vi "Tusk.Test.vi"(10 "Tusk in":refnum<class "Tusk.lvclass">) -> ()   [LabVIEW 2018, in "Application.lvlib" / "Tusk.lvclass"]
uses:
  Tusk.lvclass
  Tusk.lvclass/Tusk.ctl
  Store Class/Store.lvclass/Store.ctl
  Dictionary Class/Dictionary.lvclass/Dictionary.ctl
  Message Class/Message.lvclass/Message.ctl
  Tusk.ValidateName.vi
  Tusk.SetName (Global).vi
  Store Class/VIs/Create.vi
  Tusk.GetName (Global).vi
  Store Class/VIs/Destroy.vi
  Tusk.Init.vi
  Tusk.Register.vi
  Tusk.ValidateTusk (Local).vi
  Tusk.SetName (Local).vi
  Message Class/VIs/Wrap Message.vi
  Tusk.GetName (Local).vi
  Keywords Class/VIs/{Timeout}.vi
  Keywords Class/VIs/{Destructor}.vi
  Tusk.IsGlogalMessage.vi
  Tusk.MessageSenderCore.vi
  Tusk.GetTuskFromDictionary.vi
  Message Class/VIs/Split Message.vi
  Message Class/VIs/Get Message.vi
  Tusk.IsTopLevel.vi
  Tusk.KillAll(Local).vi
  Message Class/VIs/Unwrap Message.vi
  Keywords Class/VIs/{Self}.vi
  Tusk.KillMessageCore.vi
  Exceptions Class/VIs/Invalid Name Format.vi
  Keywords Class/VIs/{Constructor}.vi
  Tusk.GetDictionary.vi
  Tusk.Register.vi/ecdc04cd-daca-4470-8ca9-75b19434ba98.vi
  Dictionary Class/VIs/Get.vi
  Exceptions Class/VIs/Name (Local) Taken.vi
  Exceptions Class/VIs/Invalid Type.vi
  Tusk.GetTuskFromDictionary.vi/3fa77438-33e4-48e7-a501-c74b9750b9f8.vi
  Tusk.GetTuskFromDictionary.vi/bb4b4b2f-5120-4767-9776-c61ed956de36.vi
  Tusk.MessageAllSenderCore.vi
  Keywords Class/VIs/{All}.vi
  Dictionary Class/VIs/Get Data DVR.vi
  Tusk.MessageAllSenderCore.vi/1679c56e-e765-44f0-aff8-f47c4dbf3d60.vi
  <vilib>/Utility/error.llb/Trim Whitespace.vi
  Dictionary Class/VIs/Create.vi
  Dictionary Class/VIs/Destroy.vi
  Tusk.TuskBox.vi
  <vilib>/Utility/error.llb/Error Cluster From Error Code.vi
  <vilib>/Utility/SystemLogging/Write to System Log.vi
  Store Class/Store.lvclass
  Dictionary Class/Dictionary.lvclass
  Message Class/Message.lvclass
panel:
  out "x-y":dbl format="%^#_6e"
  out "Recieved Message":string
  in  "Send":bool
  in  "Message":string="Hello World!"
  in  "stop":bool
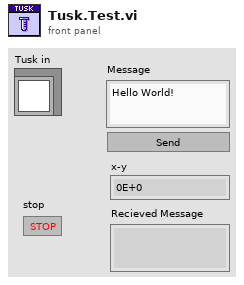
[diagram p1: front panel]
types:
  T1 = typedef "Application.lvlib/Message.lvclass/Event Registration Refnum.ctl" = refnum<event-registration>
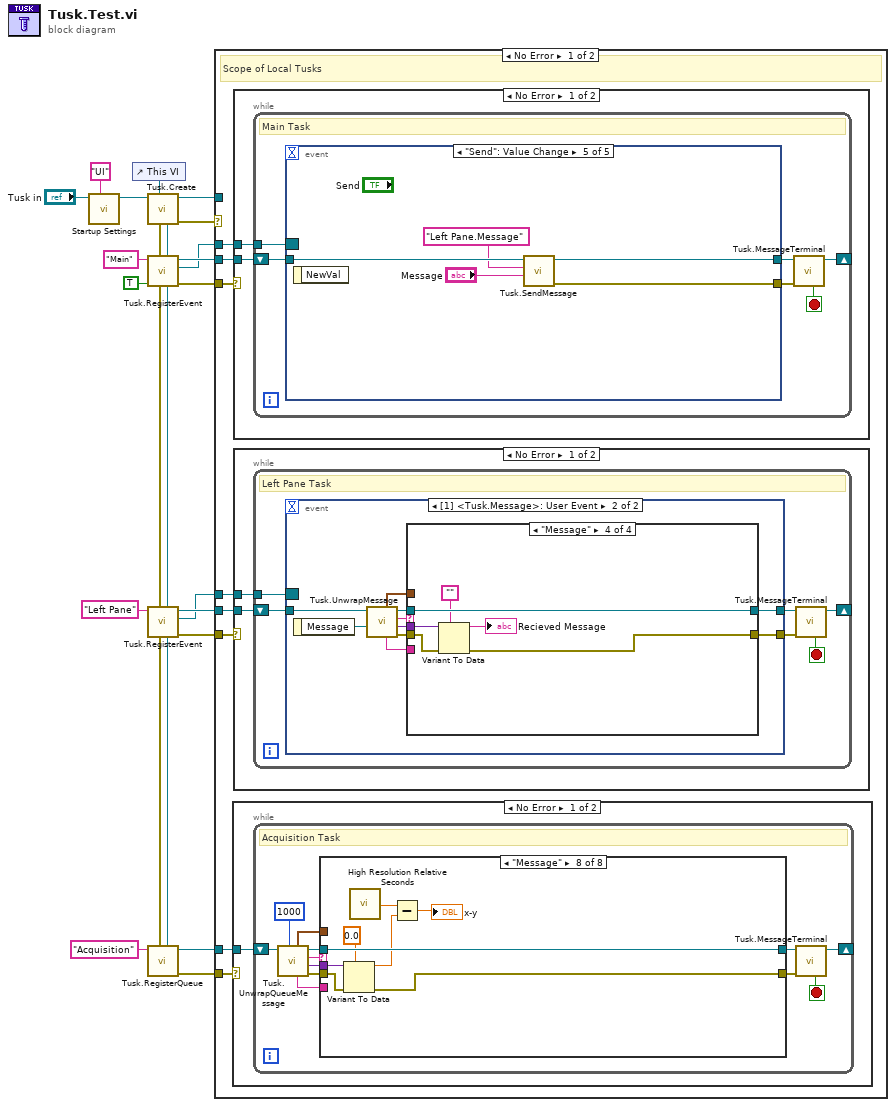
[diagram p0: block diagram]
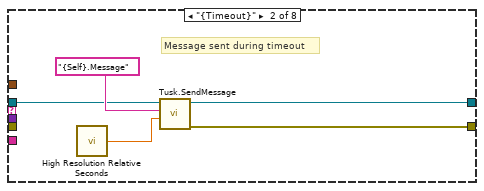
[diagram p3: hidden frame]
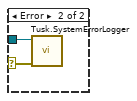
[diagram p9: hidden frame]
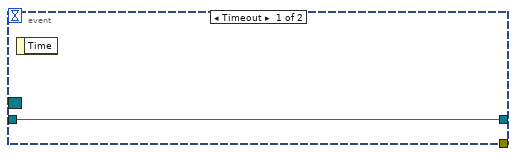
[diagram p10: hidden frame]
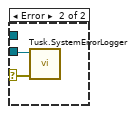
[diagram p14: hidden frame]
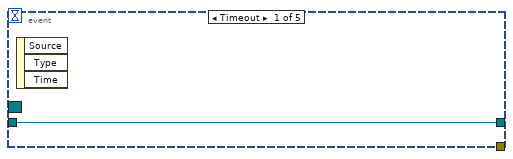
[diagram p15: hidden frame]
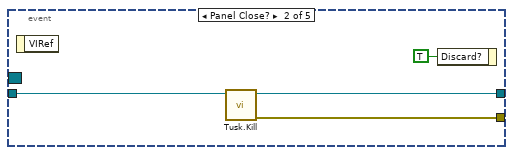
[diagram p16: hidden frame]
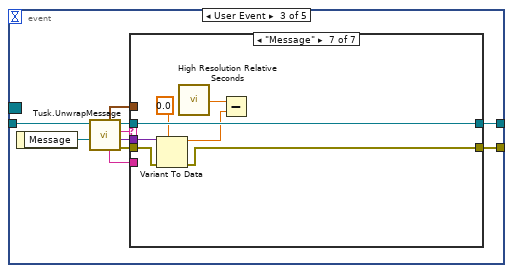
[diagram p17: hidden frame]
diagram:
  n1 = call "Startup Settings.vi"("Name(Global)"="UI", "Tusk in"="Tusk in") -> ("Tusk out"=w4:refnum<class "Tusk.lvclass">)  [unwired: 8 in, 1 out]
  n2 = control-ref of="This VI"() -> (w13:refnum<vi>)
  n3 = call "Tusk.Create.vi"("This VI"=w13, "Tusk in"=w4) -> ("error out"=w2:errorcluster, "Tusk out"=w1:refnum<class "Tusk.lvclass">, "Tusk out (copy)"=w23:refnum<class "Tusk.lvclass">, "error out (copy)"=w24:errorcluster)  [unwired: 6 in]
  n4 = call "Tusk.RegisterEvent.vi"("Tusk in"=w23, "error in (no error)"=w24, "Top Level?"=TRUE, "Name (Local)"="Main" ("Name")) -> ("error out"=w22:errorcluster, "Message Event Reg Ref"=w14:T1, "Tusk out"=w21:refnum<class "Tusk.lvclass">, "Tusk out (copy)"=w18:refnum<class "Tusk.lvclass">, "error out (copy)"=w19:errorcluster)  [unwired: 3 in]
  n5 = call "Tusk.RegisterEvent.vi"("Tusk in"=w18, "error in (no error)"=w19, "Name (Local)"="Left Pane" ("Name")) -> ("error out"=w17:errorcluster, "Message Event Reg Ref"=w11:T1, "Tusk out"=w20:refnum<class "Tusk.lvclass">, "Tusk out (copy)"=w9:refnum<class "Tusk.lvclass">, "error out (copy)"=w10:errorcluster)  [unwired: 4 in]
  n6 = call "Tusk.RegisterQueue.vi"("Tusk in"=w9, "error in (no error)"=w10, "Name(Local)"="Acquisition" ("Name")) -> ("error out"=w8:errorcluster, "Tusk out"=w6:refnum<class "Tusk.lvclass">)  [unwired: 5 in, 2 out]
  n7 = case shown="No Error" w2 {
    selector: w2 -> [_ w158]
    tunnel: w22 -> [w32 _]
    tunnel: w21 -> [w31 _]
    tunnel: w20 -> [w30 _]
    tunnel: w17 -> [w29 _]
    tunnel: w14 -> [w28 _]
    tunnel: w11 -> [w27 _]
    tunnel: w8 -> [w26 _]
    tunnel: w6 -> [w25 _]
    tunnel: w1 -> [_ w159]
    frame No Error {
      # "Scope of Local Tusks"
      n8 = case shown="No Error" w26 {
        selector: w26 -> [_ w71]
        tunnel: w25 -> [w33 w72]
        frame No Error {
          n9 = while {
            shift-right: [w45] -> _
            shift-left: w33 -> [w44]
            stop <- w40 stop-if-true
            # "Acquisition Task"
            n10 = call "Tusk.UnwrapQueueMessage.vi"("timeout in ms (-1)"=1000, "Tusk in"=w44) -> ("error out"=w42:errorcluster, "Data"=w38:variant, "Message"=w39:string, "Tusk out"=w43:refnum<class "Tusk.lvclass">, "Sender"=w36:string, "Time Sent"=w37:timestamp)  [unwired: 4 in]
            n11 = case shown="\"Message\"" w39 {
              tunnel: w42 -> [w46 _ w53 w55 w57 w59 w61 w66]
              tunnel: w43 -> [w47 w50 w54 w56 w58 w60 w62 w70]
              tunnel: [w47 w49 w54 w56 w58 w60 w62 w70] -> w41
              tunnel: [w46 w48 w53 w55 w57 w59 w61 w64] -> w35
              tunnel: w38 -> [_ _ _ _ _ _ _ w65]
              tunnel: w37 -> [_ _ _ _ _ _ _ _]
              tunnel: w36 -> [_ _ _ _ _ _ _ _]
              frame Default {
              }
              frame "{Timeout}" {
                # "Message sent during timeout"
                n12 = call <vilib>:"High Resolution Relative Seconds.vi"() -> ("relative seconds"=w51:dbl)
                n13 = call "Tusk.SendMessage.vi"("Data"=w51, "Local Tusk.Message / Global Tusk.Local Tusk. Message"="{Self}.Message", "Tusk in"=w50) -> ("error out"=w48:errorcluster, "Tusk out"=w49:refnum<class "Tusk.lvclass">)  [unwired: 7 in]
              }
              frame "{Constructor}" {
                # "Called at successful creation of a local Tusk"
              }
              frame "{Destructor}" {
                # "Last message called before local Tusk is destroyed"
              }
              frame "{!Private Message}" {
                # "Private messages are are scoped to the {Self} Tusk"
              }
              frame "{#Protected Message}" {
                # "Protected messages are are scoped to the Tusks in the\nVI"
              }
              frame "Public Message" {
                # "Public messages are are scoped to all Tusks globally"
              }
              frame "Message" {
                n14 = Variant To Data(error in=w66, type=0.0 ("x-y"), Variant=w65) -> (data=w67:dbl, error out=w64:errorcluster)
                n15 = call <vilib>:"High Resolution Relative Seconds.vi"() -> ("relative seconds"=w68:dbl)
                n16 = Subtract(x=w68, y=w67) -> (x-y=→"x-y":dbl)
              }
            }
            n17 = call "Tusk.MessageTerminal.vi"("error in (no error)"=w35, "Tusk in"=w41) -> ("Tusk out"=w45:refnum<class "Tusk.lvclass">, "Stop?"=w40:bool)  [unwired: 8 in]
          }
        }
        frame Error {
          n18 = call "Tusk.SystemErrorLogger.vi"("error in (no error)"=w71, "Tusk in"=w72) -> ()  [unwired: 8 in, 2 out]
        }
      }
      n19 = case shown="No Error" w32 {
        selector: w32 -> [_ w156]
        tunnel: w31 -> [w107 w157]
        tunnel: w28 -> [w106 _]
        frame No Error {
          n20 = while {
            shift-right: [w109] -> _
            shift-left: w107 -> [w113]
            tunnel: w106 -> [w112]
            stop <- w108 stop-if-true
            # "Main Task"
            n21 = event shown="[4] \"Send\": Value Change" {
              selector: w112 -> [_ _ _ _ _]
              dyn-events: _ -> [_ _ _ _ _]
              timeout: _ -> [_ _ _ _ _]
              tunnel: w113 -> [w114 w117 w128 w150 w155]
              tunnel: [w114 w115 w121 w149 w154] -> w111
              tunnel: [_ w116 w120 w148 w152] -> w110
              event Timeout {
                n22 = event-data() -> ()  [unwired: 1 in, 3 out]
              }
              event Panel Close? {
                n23 = event-data() -> ()  [unwired: 1 in, 1 out]
                n24 = call "Tusk.Kill.vi"("Tusk in"=w117) -> ("error out"=w116:errorcluster, "Tusk out"=w115:refnum<class "Tusk.lvclass">)  [unwired: 9 in]
                n25 = event-data("Discard?"=TRUE) -> ()  [unwired: 1 in, 1 out]
              }
              event User Event {
                n26 = event-data() -> ("Message"=w119:refnum<class "Message.lvclass">)  [unwired: 1 in]
                n27 = call "Tusk.UnwrapMessage.vi"("Message"=w119, "Tusk in"=w128) -> ("error out"=w127:errorcluster, "Data"=w122:variant, "Message"=w126:string, "Tusk out"=w125:refnum<class "Tusk.lvclass">, "Sender"=w124:string, "Time Sent"=w123:timestamp)  [unwired: 4 in]
                n28 = case shown="\"Message\"" w126 {
                  tunnel: w127 -> [w129 w131 w133 w135 w137 w139 w142]
                  tunnel: w125 -> [w130 w132 w134 w136 w138 w140 w147]
                  tunnel: w124 -> [_ _ _ _ _ _ _]
                  tunnel: w123 -> [_ _ _ _ _ _ _]
                  tunnel: w122 -> [_ _ _ _ _ _ w143]
                  tunnel: [w130 w132 w134 w136 w138 w140 w147] -> w121
                  tunnel: [w129 w131 w133 w135 w137 w139 w141] -> w120
                  frame Default {
                  }
                  frame "{Constructor}" {
                    # "Called at successful creation of a local Tusk"
                  }
                  frame "{Destructor}" {
                    # "Last message called before local Tusk is destroyed"
                  }
                  frame "{!Private Message}" {
                    # "Private messages are are scoped to the {Self} Tusk"
                  }
                  frame "{#Protected Message}" {
                    # "Protected messages are are scoped to the Tusks in the\nVI"
                  }
                  frame "Public Message" {
                    # "Public messages are are scoped to all Tusks globally"
                  }
                  frame "Message" {
                    n29 = Variant To Data(error in=w142, type=0.0 ("x-y"), Variant=w143) -> (data=w144:dbl, error out=w141:errorcluster)
                    n30 = call <vilib>:"High Resolution Relative Seconds.vi"() -> ("relative seconds"=w145:dbl)
                    n31 = Subtract(x=w145, y=w144) -> ()  [unwired: 1 out]
                  }
                }
              }
              event "stop": Value Change {
                n32 = event-data() -> ()  [unwired: 1 in, 1 out]
                n33 = call "Tusk.Kill.vi"("Tusk in"=w150) -> ("error out"=w148:errorcluster, "Tusk out"=w149:refnum<class "Tusk.lvclass">)  [unwired: 9 in]
              }
              event "Send": Value Change {
                n34 = event-data() -> ()  [unwired: 1 in, 1 out]
                n35 = call "Tusk.SendMessage.vi"("Data"="Message", "Local Tusk.Message / Global Tusk.Local Tusk. Message"="Left Pane.Message", "Tusk in"=w155) -> ("error out"=w152:errorcluster, "Tusk out"=w154:refnum<class "Tusk.lvclass">)  [unwired: 7 in]
              }
            }
            n36 = call "Tusk.MessageTerminal.vi"("error in (no error)"=w110, "Tusk in"=w111) -> ("Tusk out"=w109:refnum<class "Tusk.lvclass">, "Stop?"=w108:bool)  [unwired: 8 in]
          }
        }
        frame Error {
          n37 = call "Tusk.SystemErrorLogger.vi"("error in (no error)"=w156, "Tusk in"=w157) -> ()  [unwired: 8 in, 2 out]
        }
      }
      n38 = case shown="No Error" w29 {
        selector: w29 -> [_ w104]
        tunnel: w30 -> [w74 w105]
        tunnel: w27 -> [w73 _]
        frame No Error {
          n39 = while {
            shift-right: [w77] -> _
            shift-left: w74 -> [w80]
            tunnel: w73 -> [w79]
            stop <- w75 stop-if-true
            # "Left Pane Task"
            n40 = event shown="[1] <Tusk.Message>: User Event" {
              selector: w79 -> [_ _]
              dyn-events: _ -> [_ _]
              timeout: _ -> [_ _]
              tunnel: w80 -> [w81 w85]
              tunnel: [w81 w84] -> w78
              tunnel: [_ w83] -> w76
              event Timeout {
                n41 = event-data() -> ()  [unwired: 1 in, 1 out]
              }
              event User Event {
                n42 = event-data() -> ("Message"=w82:refnum<class "Message.lvclass">)  [unwired: 1 in]
                n43 = call "Tusk.UnwrapMessage.vi"("Message"=w82, "Tusk in"=w85) -> ("error out"=w91:errorcluster, "Data"=w86:variant, "Message"=w90:string, "Tusk out"=w89:refnum<class "Tusk.lvclass">, "Sender"=w88:string, "Time Sent"=w87:timestamp)  [unwired: 4 in]
                n44 = case shown="\"Message\"" w90 {
                  tunnel: w91 -> [w92 w94 w96 w102]
                  tunnel: w89 -> [w93 w95 w97 w103]
                  tunnel: w88 -> [_ _ _ _]
                  tunnel: w87 -> [_ _ _ _]
                  tunnel: w86 -> [_ _ _ w101]
                  tunnel: [w93 w95 w97 w103] -> w84
                  tunnel: [w92 w94 w96 w98] -> w83
                  frame Default {
                  }
                  frame "{Constructor}" {
                  }
                  frame "{Destructor}" {
                  }
                  frame "Message" {
                    n45 = Variant To Data(error in=w102, type="", Variant=w101) -> (data=→"Recieved Message":string, error out=w98:errorcluster)
                  }
                }
              }
            }
            n46 = call "Tusk.MessageTerminal.vi"("error in (no error)"=w76, "Tusk in"=w78) -> ("Tusk out"=w77:refnum<class "Tusk.lvclass">, "Stop?"=w75:bool)  [unwired: 8 in]
          }
        }
        frame Error {
          n47 = call "Tusk.SystemErrorLogger.vi"("error in (no error)"=w104, "Tusk in"=w105) -> ()  [unwired: 8 in, 2 out]
        }
      }
    }
    frame Error {
      # "Error case at failure start Tusk (Errors are recorded at the Event Viewer)"
      n48 = call "Tusk.SystemErrorLogger.vi"("error in (no error)"=w158, "Tusk in"=w159) -> ()  [unwired: 8 in, 2 out]
    }
  }
